vi "Shutdown - OLD.vi"(0 "Limits File":path, 5 "Results File":path, 11 "error in":errorcluster) -> (4 "Results Data Array":string[][](array[string]), 15 "error out":errorcluster)   [LabVIEW 2024]
doc: "Fake shutdown test"
uses:
  <userlib>/_OpenG.lib/time/time.llb/openg_time.lvlib
  <userlib>/_OpenG.lib/appcontrol/appcontrol.llb/openg_application_control.lvlib
  I2C/libMPSSE-I2C.lvlib
panel:
  # "Shutdown Test"
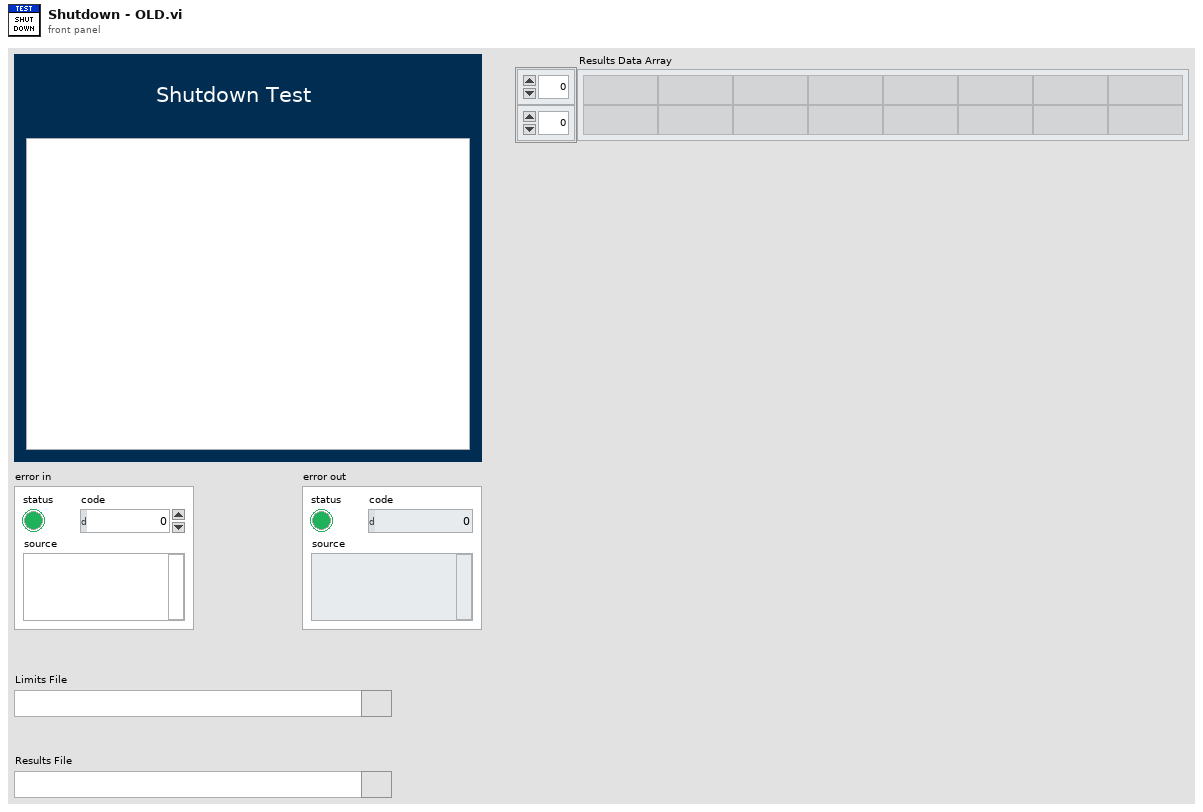
[diagram p1: front panel]
types:
  T1 = typedef "FGV - Enum" = enum16{"Cleanup", "Get Data", "Open UDP", "Initialise DAQ", "Initialise I2C"}
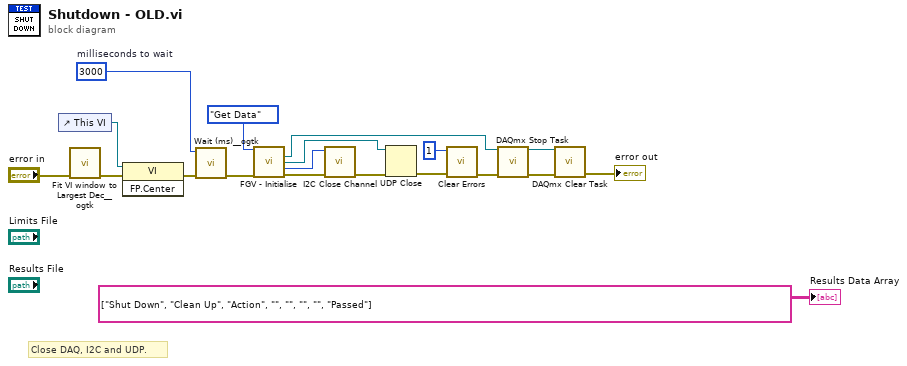
[diagram p0: block diagram]
diagram:
  w18 = u32 3000  # milliseconds to wait
  # "Close DAQ, I2C and UDP."
  n1 = control-ref of="This VI"() -> (w15:refnum<vi>)
  n2 = call <userlib>:"Fit VI window to Largest Dec__ogtk.vi"("error in (no error)"="error in") -> ("error out"=w17:errorcluster)  [unwired: 5 in, 1 out]
  n3 = invoke class="VI" method="FP.Center"(reference=w15, error in=w17) -> (error out=w16:errorcluster)  [unwired: 1 in, 2 out]
  n4 = call <userlib>:"Wait (ms)__ogtk.vi"("error in (no error)"=w16, "milliseconds to wait"=w18) -> ("error out"=w12:errorcluster)  [unwired: 8 in, 1 out]
  n5 = call "FGV - Initialise.vi"("Enum"=FGV_-_Enum."Get Data", "Error In"=w12) -> ("task out"=w7:refnum<k21>, "connection ID"=w8:refnum<k16>, "Handle Out"=w9:u64, "Error Out"=w10:errorcluster)  [unwired: 10 in]
  n6 = call "I2C Close Channel.vi"("error in (no error)"=w10, "handle"=w9) -> ("error out"=w5:errorcluster)  [unwired: 7 in, 2 out]
  n7 = UDP Close(connection ID=w8, 8:w5) -> (error out=w4:errorcluster)  [unwired: 1 out]
  n8 = call <vilib>:"Clear Errors.vi"("error in (no error)"=w4, "specific error code to clear (0: all)"=1) -> ("error out"=w3:errorcluster)  [unwired: 4 in, 1 out]
  n9 = call <vilib>:"DAQmx Stop Task.vi"("task/channels in"=w7, "error in"=w3) -> ("task out"=w13:refnum<k21>, "error out"=w14:errorcluster)  [unwired: 12 in]
  n10 = call <vilib>:"DAQmx Clear Task.vi"("task in"=w13, "error in"=w14) -> ("error out"=→"error out":errorcluster)  [unwired: 13 in]
  "Results Data Array" <- string[][] [["Shut Down", "Clean Up", "Action", "", "", "", "", "Passed"]]
